vi "histo_qm_d@16.vi"(10 "Histo (e)":T2, 11 "Pièce":T1) -> (2 "Histo (s)":T2)   [LabVIEW 2010, in "lv_07.lvlib"]
doc: "Si le tableau Qper des consommations est saisi, on calcule la moyenne et l'écart-type."
uses:
  lv_07.lvlib
  c_histo.ctl
  c_pi_wilson.ctl
  <vilib>/Analysis/NI_AALBase.lvlib
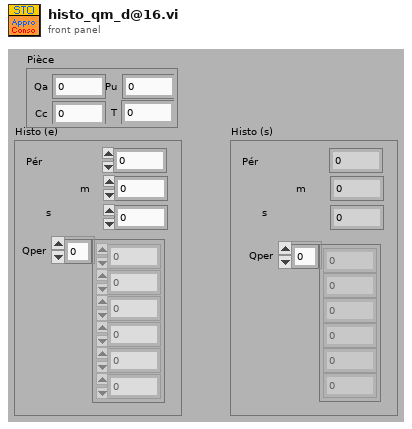
[diagram p1: front panel]
types:
  T1 = typedef "lv_07.lvlib/c_pi_wilson.ctl" = cluster{"T":dbl, "Pu":dbl, "Qa":dbl, "Cc":dbl}
  T2 = typedef "lv_07.lvlib/c_histo.ctl" = cluster{"Pér":dbl, "Qper":dbl[], "s":dbl, "m":dbl}
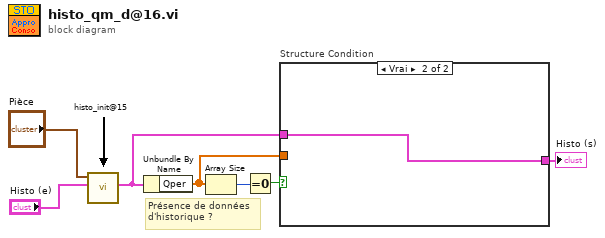
[diagram p0: block diagram]
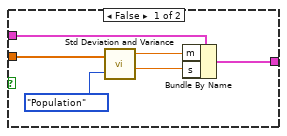
[diagram p2: hidden frame]
diagram:
  # "Présence de données\nd'historique ?"
  n1 = call "histo_init@15.vi"("Histo (e)"="Histo (e)", "Pièce"="Pièce") -> ("Histo (s)"=w1:T2)  [unwired: 7 in]
  n2 = Unbundle By Name(w1) -> ("Qper"=w6:dbl[])
  n3 = Array Size(array=w6) -> (size(s)=w4:i32)
  n4 = Equal To 0?(x=w4) -> (x = 0?=w5:bool)
  n5 = case "Structure Condition" shown="Vrai" w5 {
    tunnel: w1 -> [w12 w14]
    tunnel: w6 -> [w13 _]
    tunnel: [w8 w14] -> w7
    frame False {
      n6 = call <vilib>:"Std Deviation and Variance.vi"("X"=w13, "Weighting (Sample)"=enum16{"Sample", "Population"}."Population") -> ("mean"=w11:dbl, "standard deviation"=w10:dbl)  [unwired: 1 out]
      n7 = Bundle By Name(cluster=w12, "m"=w11, "s"=w10) -> (w8:T2)
    }
    frame True {
    }
  }
  "Histo (s)" <- w7
